vi "Update Guest Name.vi"(0 "Rooms Manager Model in":refnum<class "Rooms Manager Model.lvclass">, 5 "IsAvailable":bool, 7 "Guest Name":string, 11 "error in (no error)":errorcluster) -> (4 "Rooms Manager Model out":refnum<class "Rooms Manager Model.lvclass">, 15 "error out":errorcluster)   [LabVIEW 2023, in "Rooms Manager Model.lvlib" / "Rooms Manager Model.lvclass"]
uses:
  Rooms Manager Model.lvclass
  Rooms Manager Model.lvclass/Rooms Manager Model.ctl
  Guest Manager Model/Guest Manager Model Messages/Update Guest Name Msg/Update Guest Name Msg.lvclass
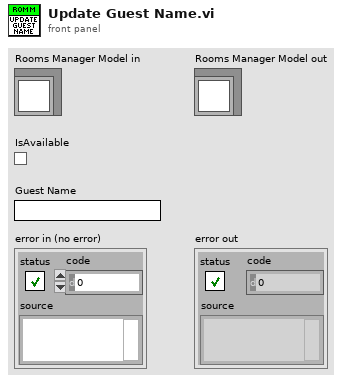
[diagram p1: front panel]
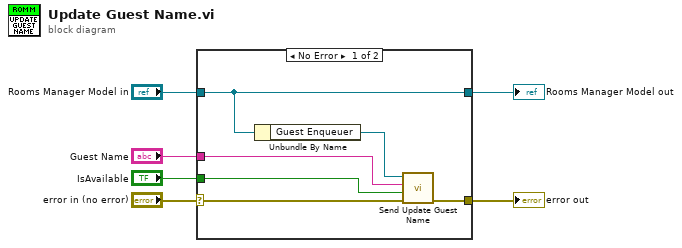
[diagram p0: block diagram]
diagram:
  n1 = case shown="No Error" "error in (no error)" {
    selector: "error in (no error)" -> [w12 w14]
    tunnel: [w11 w14] -> w5
    tunnel: [w10 w13] -> w3
    tunnel: "Rooms Manager Model in" -> [w10 w13]
    tunnel: "Guest Name" -> [w8 _]
    tunnel: "IsAvailable" -> [w7 _]
    frame No Error {
      n2 = Unbundle By Name(w10) -> ("Guest Enqueuer"=w9:refnum<class "Message Enqueuer.lvclass">)
      n3 = call "Send Update Guest Name.vi"("error in (no error)"=w12, "IsAvailable"=w7, "Guest Name"=w8, "Message Enqueuer"=w9) -> ("error out"=w11:errorcluster)  [unwired: 6 in, 1 out]
    }
    frame Error {
    }
  }
  "error out" <- w5
  "Rooms Manager Model out" <- w3
